vi "Interpolate Parameter.vi"(8 "error in (no error)":errorcluster, 9 "Fake Point":dbl, 10 "Parameter-array":dbl[](array[numeric]) format="%.2p", 11 "XY-data":cluster{"X-array":dbl[], "Y-array":dbl[]}[](array[cluster]) {"Y-array" format="%.2p"; "X-array" format="%.2p"}) -> (0 "error out":errorcluster, 2 "Interpolated Parameter-array":dbl[](array[numeric]), 3 "Interpolated XY-data out":cluster{"X-array":dbl[], "Y-array":dbl[]}[](array[cluster]) {"Y-array" format="%.2p"; "X-array" format="%.2p"})   [LabVIEW 2019, in "xy_utilities.lvlib"]
doc: "Interpolate the input <b>XY-data</b> along the <b>Parameter-array</b> axis."
uses:
  xy_utilities.lvlib
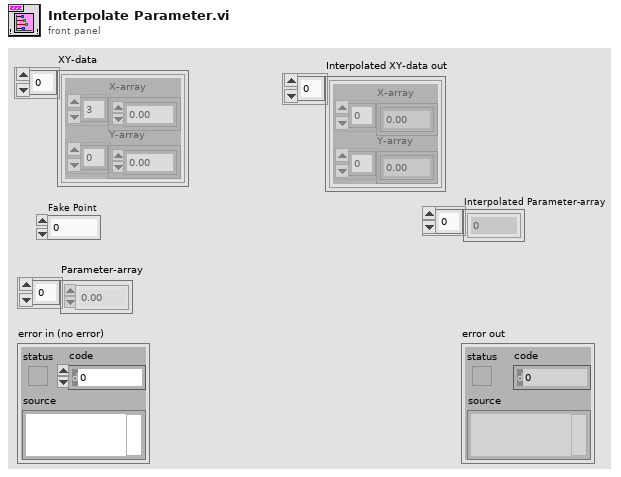
[diagram p1: front panel]
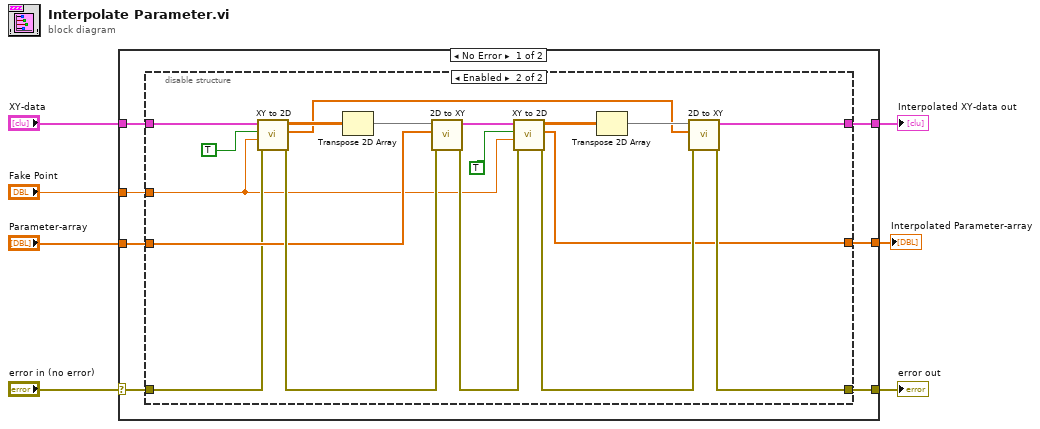
[diagram p0: block diagram]
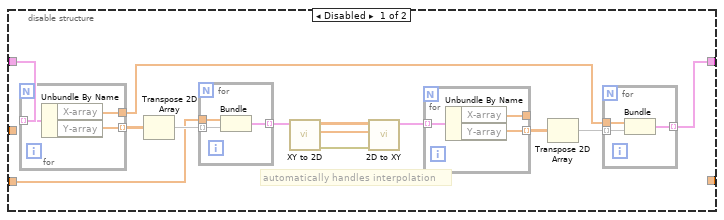
[diagram p2: hidden frame]
diagram:
  n1 = case shown="No Error" "error in (no error)" {
    selector: "error in (no error)" -> [w12 w60]
    tunnel: "XY-data" -> [w11 w59]
    tunnel: [w10 w59] -> w5
    tunnel: [w8 w60] -> w4
    tunnel: "Parameter-array" -> [w13 w58]
    tunnel: [w9 w58] -> w3
    tunnel: "Fake Point" -> [w14 _]
    frame No Error {
      n2 = disable-structure shown="Enabled" {
        disable-tunnel: w11 -> [w17 w41]
        disable-tunnel: w14 -> [_ w46]
        disable-tunnel: w13 -> [w16 w48]
        disable-tunnel: w12 -> [_ w47]
        disable-tunnel: [_ w44] -> w8
        disable-tunnel: [w15 w43] -> w10
        disable-tunnel: [_ w42] -> w9
        frame Disabled {
          # "automatically handles interpolation"
          n3 = for {
            tunnel: w17 -> [w39] mode=indexing
            tunnel: [w38] -> w27 mode=indexing
            tunnel: [w37] -> w23
            n4 = Unbundle By Name(w39) -> ("X-array"=w37:dbl[], "Y-array"=w38:dbl[])
          }
          n5 = Transpose 2D Array(2D array=w27) -> (transposed array=w26:dbl[][])
          n6 = for {
            tunnel: w26 -> [w36] mode=indexing
            tunnel: w16 -> [w35]
            tunnel: [w34] -> w19 mode=indexing
            n7 = Bundle("Parameter-array"=w35, w36) -> (w34:cluster{"Parameter-array":dbl[], dbl[]})  [unwired: 1 in]
          }
          n8 = call "XY to 2D.vi"("XY-data"=w19) -> ("error out"=w20:errorcluster, "X Array"=w21:dbl[], "2D Z Array"=w22:dbl[][])  [unwired: 7 in, 1 out]
          n9 = call "2D to XY.vi"("error in (no error)"=w20, "X Array"=w21, "2D Z Array"=w22) -> ("XY-data out"=w18:cluster{"X-array":dbl[], "Y-array":dbl[]}[])  [unwired: 7 in, 1 out]
          n10 = for {
            tunnel: w18 -> [w33] mode=indexing
            tunnel: [w32] -> w24 mode=indexing
            tunnel: [w31] -> _
            n11 = Unbundle By Name(w33) -> ("X-array"=w31:dbl[], "Y-array"=w32:dbl[])
          }
          n12 = Transpose 2D Array(2D array=w24) -> (transposed array=w25:dbl[][])
          n13 = for {
            tunnel: w25 -> [w30] mode=indexing
            tunnel: w23 -> [w29]
            tunnel: [w28] -> w15 mode=indexing
            n14 = Bundle("X-array"=w29, w30) -> (w28:cluster{"X-array":dbl[], dbl[]})  [unwired: 1 in]
          }
        }
        frame Enabled {
          n15 = call "XY to 2D.vi"("error in (no error)"=w47, "Fake Point"=w46, "Interpolate [T]"=TRUE, "XY-data"=w41) -> ("error out"=w50:errorcluster, "X Array"=w40:dbl[], "2D Z Array"=w51:dbl[][])  [unwired: 4 in, 1 out]
          n16 = Transpose 2D Array(2D array=w51) -> (transposed array=w52:dbl[][])
          n17 = call "2D to XY.vi"("error in (no error)"=w50, "X Array"=w48, "2D Z Array"=w52) -> ("error out"=w56:errorcluster, "XY-data out"=w53:cluster{"X-array":dbl[], "Y-array":dbl[]}[])  [unwired: 7 in]
          n18 = call "XY to 2D.vi"("error in (no error)"=w56, "Fake Point"=w46, "Interpolate [T]"=TRUE, "XY-data"=w53) -> ("error out"=w54:errorcluster, "X Array"=w42:dbl[], "2D Z Array"=w57:dbl[][])  [unwired: 4 in, 1 out]
          n19 = Transpose 2D Array(2D array=w57) -> (transposed array=w55:dbl[][])
          n20 = call "2D to XY.vi"("error in (no error)"=w54, "X Array"=w40, "2D Z Array"=w55) -> ("error out"=w44:errorcluster, "XY-data out"=w43:cluster{"X-array":dbl[], "Y-array":dbl[]}[])  [unwired: 7 in]
        }
      }
    }
    frame Error {
    }
  }
  "error out" <- w4
  "Interpolated XY-data out" <- w5
  "Interpolated Parameter-array" <- w3
